vi "Register For User Event.vi"(8 "Error In":errorcluster, 11 "User Event Reference":T2) -> (0 "Error Out":errorcluster, 3 "User Event Registration Reference":T1)   [LabVIEW 2023, in "QSM - IODocs.lvlib"]
doc: "This VI registers for the user event for the Queued Message Handler template."
uses:
  QSM - IODocs.lvlib
  Controls/User Event Reference.ctl
  Controls/User Event Registration Reference.ctl
  Controls/Event Handler Message.ctl
  Controls/User Event Type.ctl
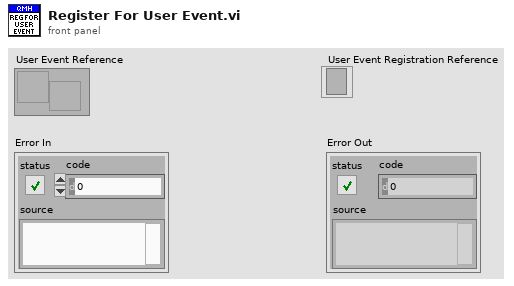
[diagram p1: front panel]
types:
  T1 = typedef "QSM - IODocs.lvlib/User Event Registration Reference.ctl" = refnum<event-registration>
  T2 = typedef "QSM - IODocs.lvlib/User Event Reference.ctl" = refnum<user-event>
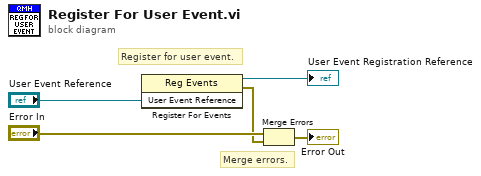
[diagram p0: block diagram]
diagram:
  # "Merge errors."
  # "Register for user event."
  n1 = register-events("User Event Reference") -> (reference out=→"User Event Registration Reference":refnum<event-registration>, error out=w2:errorcluster)  [unwired: 2 in]
  n2 = Merge Errors("Error In", w2) -> (→"Error Out":errorcluster)
